vi "abortDynVi.vi"(8 "error in (no error)":errorcluster, 11 "Handler.UserEvent.Console in":refnum<class "Handler.UserEvent.Console.lvclass">) -> (0 "error out":errorcluster, 3 "Handler.UserEvent.Console out":refnum<class "Handler.UserEvent.Console.lvclass">)   [LabVIEW 2017, in "Error Log.lvlib" / "Handler.UserEvent.Console.lvclass"]
doc: "Kill dynamic VI if necessary."
uses:
  Handler.UserEvent.Console.lvclass
  Handler.UserEvent.Console.lvclass/Handler.UserEvent.Console.ctl
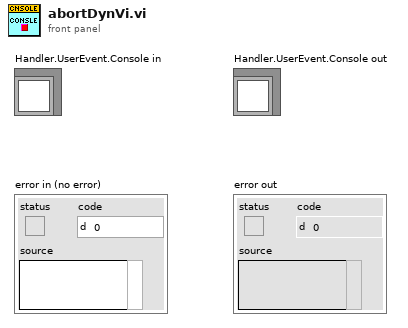
[diagram p1: front panel]
types:
  T1 = enum32{"Bad", "Idle", "Run top level", "Running"}
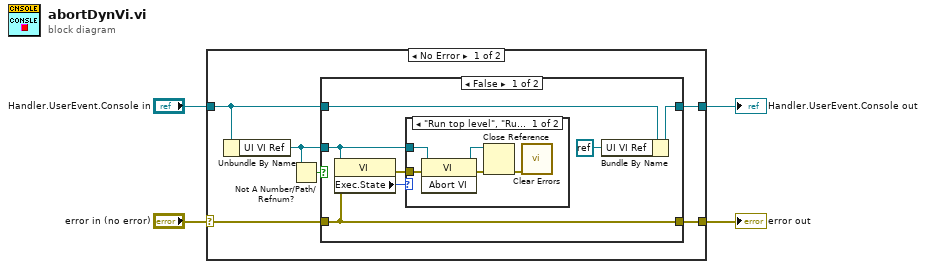
[diagram p0: block diagram]
diagram:
  n1 = case shown="No Error" "error in (no error)" {
    selector: "error in (no error)" -> [w6 w26]
    tunnel: [w5 w26] -> w3
    tunnel: [w9 w25] -> w1
    tunnel: "Handler.UserEvent.Console in" -> [w10 w25]
    frame No Error {
      n2 = Unbundle By Name(w10) -> ("UI VI Ref"=w8:refnum<vi>)
      n3 = Not A Number/Path/Refnum?(number/path/refnum=w8) -> (NaN/Path/Refnum?=w7:bool)
      n4 = case shown="False" w7 {
        tunnel: w10 -> [w17 w23]
        tunnel: [w15 w23] -> w9
        tunnel: w6 -> [w11 w24]
        tunnel: w8 -> [w12 _]
        tunnel: [w11 w24] -> w5
        frame False {
          n5 = property class="VI"(reference=w12, error in=w11) -> (error out=w13:errorcluster, "Exec.State"=w16:T1)  [unwired: 1 out]
          n6 = case shown="\"Run top level\", \"Running\"" w16 {
            tunnel: w12 -> [w20 _]
            tunnel: w13 -> [w18 _]
            frame "Run top level", "Running" {
              n7 = invoke class="VI" method="Abort VI"(reference=w20, error in=w18) -> (reference out=w19:refnum<vi>, error out=w22:errorcluster)  [unwired: 1 in, 1 out]
              n8 = Close Reference(reference=w19, error in (no error)=w22) -> (error out=w21:errorcluster)
              n9 = call <vilib>:"Clear Errors.vi"("error in (no error)"=w21) -> ()  [unwired: 5 in, 2 out]
            }
            frame Default {
            }
          }
          n10 = Bundle By Name(cluster=w17, "UI VI Ref"=refnum<k0> refnum) -> (w15:refnum<class "Handler.UserEvent.Console.lvclass">)
        }
        frame True {
        }
      }
    }
    frame Error {
    }
  }
  "error out" <- w3
  "Handler.UserEvent.Console out" <- w1
